vi "Scanmirrors.vi"() -> ()   [LabVIEW 2010]
panel:
  in  "Y Amplitude":dbl caption="Amplitude"
  in  "X Amplitude":dbl caption="Amplitude"
  in  "stop":bool
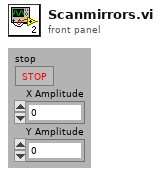
[diagram p1: front panel]
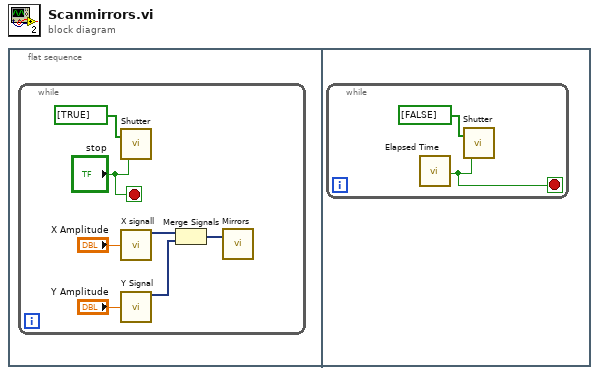
[diagram p0: block diagram]
diagram:
  n1 = flat-sequence {
    frame #0 {
      n2 = while {
        stop <- "stop" stop-if-true
        n3 = call "Shutter"("data"=bool[] [TRUE], "stop (T)"="stop") -> ()  [unwired: 16 in, 2 out]
        n4 = call "X signall"("Amplitude"="X Amplitude") -> ("Sine"=w7:dynamicdata)  [unwired: 13 in, 1 out]
        n5 = call "Y Signal"("Amplitude"="Y Amplitude") -> ("Sine"=w5:dynamicdata)  [unwired: 13 in, 1 out]
        n6 = Merge Signals(w7, w5) -> (w6:dynamicdata)
        n7 = call "Mirrors"("data"=w6) -> ()  [unwired: 17 in, 2 out]
      }
    }
    frame #1 {
      n8 = while {
        stop <- w8 stop-if-true
        n9 = call "Elapsed Time"() -> ("Time has Elapsed"=w8:bool)  [unwired: 12 in, 7 out]
        n10 = call "Shutter"("data"=bool[] [FALSE], "stop (T)"=w8) -> ()  [unwired: 16 in, 2 out]
      }
    }
  }
